vi "Event Handler.vi"(8 "error in (no error)":errorcluster, 10 "Stop Event Handler":refnum<user-event>, 11 "TreeSelection in":refnum<class "TreeSelection.lvclass">) -> (0 "error out":errorcluster)   [LabVIEW 2015, in "TreeSelection.lvclass"]
doc: "The <b>Event Handler VI</b> is a dynamic dispatch VI that should be overwritten if events are needed to create the enhanced QControl. \n\nBy inheriting from the main Control.lvclass the overwritten <b>Event Handler VI</b> will be launched asynchronously in the initialization of the QControl.\n<b> </b> <b> </b>\n©2016 Q Software Innovations, LLC (QSI)\nwritten by Quentin Alldredge\nproduced in LabVIEW 2015\n\nsupport@qsoftwareinnovations.com\nwww.qsoftwareinnovations.com\n\nAll rights reserved.\n\nRedistribution and use in source and binary forms, with or without modification, are permitted provided that the following conditions are met:\n\n * Redistributions of source code must retain the above copyright notice, this list of conditions and the following disclaimer.\n * Redistributions in binary form must reproduce the above copyright notice, this list of conditions and the following disclaimer in the documentation and/or other materials provided with the distribution.\n * Neither the name of Q Software Innovations, LLC. nor the names of its contributors may be used to endorse or promote products derived from this software without specific prior written permission.\n\nTHIS SOFTWARE IS PROVIDED BY THE COPYRIGHT HOLDERS AND CONTRIBUTORS \"AS IS\" AND ANY EXPRESS OR IMPLIED WARRANTIES, INCLUDING, BUT NOT LIMITED TO, THE IMPLIED WARRANTIES OF MERCHANTABILITY AND FITNESS FOR A PARTICULAR PURPOSE ARE DISCLAIMED. IN NO EVENT SHALL THE COPYRIGHT OWNER OR CONTRIBUTORS BE LIABLE FOR ANY DIRECT, INDIRECT, INCIDENTAL, SPECIAL, EXEMPLARY, OR CONSEQUENTIAL DAMAGES (INCLUDING, BUT NOT LIMITED TO, PROCUREMENT OF SUBSTITUTE GOODS OR SERVICES; LOSS OF USE, DATA, OR PROFITS; OR BUSINESS INTERRUPTION) HOWEVER CAUSED AND ON ANY THEORY OF LIABILITY, WHETHER IN CONTRACT, STRICT LIABILITY, OR TORT (INCLUDING NEGLIGENCE OR OTHERWISE) ARISING IN ANY WAY OUT OF THE USE OF THIS SOFTWARE, EVEN IF ADVISED OF THE POSSIBILITY OF SUCH DAMAGE."
uses:
  TreeSelection.lvclass
  TreeSelection.lvclass/TreeSelection.ctl
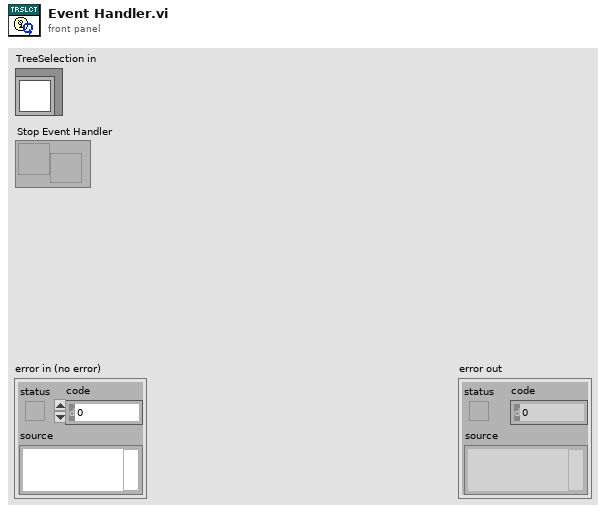
[diagram p1: front panel]
types:
  T1 = typedef "LVPoint32TypeDef.ctl" = cluster{"Horizontal":i32, "Vertical":i32}
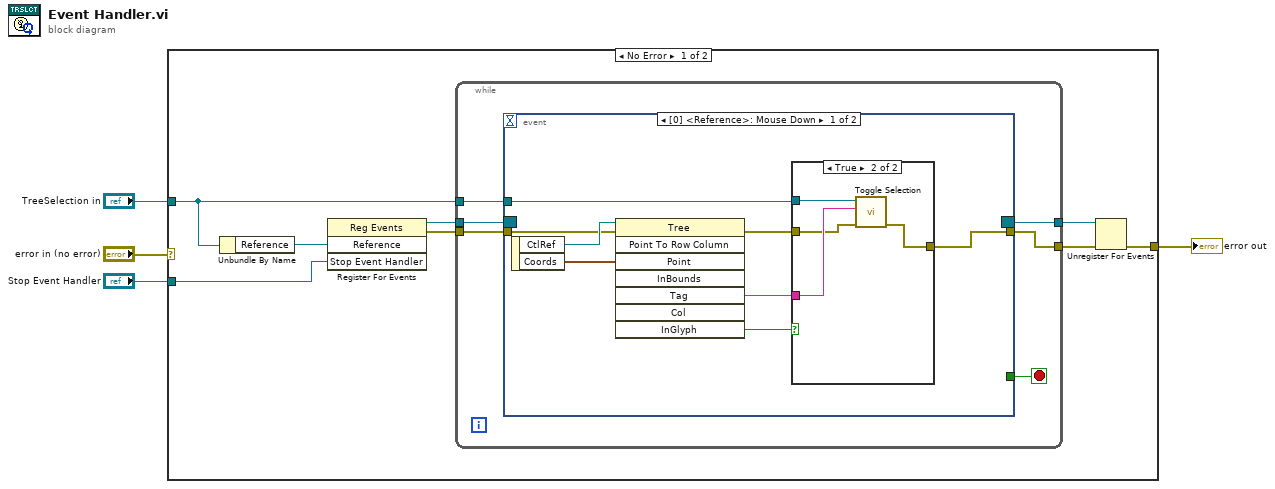
[diagram p0: block diagram]
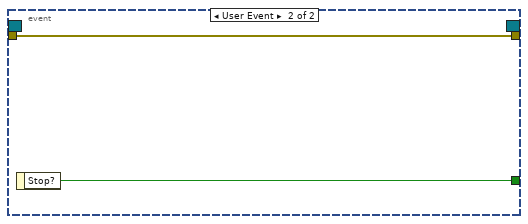
[diagram p3: hidden frame]
diagram:
  n1 = case shown="No Error" "error in (no error)" {
    selector: "error in (no error)" -> [_ w34]
    tunnel: [w9 w34] -> w3
    tunnel: "TreeSelection in" -> [w7 _]
    tunnel: "Stop Event Handler" -> [w5 _]
    frame No Error {
      n2 = Unbundle By Name(w7) -> ("Reference"=w6:refnum<vi>)
      n3 = register-events(w6, w5) -> (reference out=w12:refnum<event-registration>, error out=w11:errorcluster)  [unwired: 2 in]
      n4 = while {
        tunnel: w12 -> [w18]
        tunnel: w11 -> [w16]
        tunnel: [w15] -> w10
        tunnel: [w13] -> w8
        tunnel: w7 -> [w17]
        stop <- w14 stop-if-true
        n5 = event shown="[0] <Reference>: Mouse Down" {
          selector: w18 -> [_ _]
          dyn-events: [_ _] -> w13
          timeout: _ -> [_ _]
          tunnel: w17 -> [w24 _]
          tunnel: w16 -> [w21 w33]
          tunnel: [w19 w33] -> w15
          tunnel: [_ w32] -> w14
          event Mouse Down {
            n6 = event-data() -> ("CtlRef"=w26:refnum<vi>, "Coords"=w25:T1)  [unwired: 1 in]
            n7 = invoke class="Tree" method="Point To Row Column"(reference=w26, error in=w21, "Point"=w25) -> (error out=w20:errorcluster, "Tag"=w23:string, "InGlyph"=w22:bool)  [unwired: 5 in, 5 out]
            n8 = case shown="True" w22 {
              tunnel: w24 -> [_ w30]
              tunnel: w23 -> [_ w31]
              tunnel: w20 -> [w27 w29]
              tunnel: [w27 w28] -> w19
              frame False {
              }
              frame True {
                n9 = call-dynamic "Toggle Selection.vi"("error in (no error)"=w29, "Tag"=w31, "TreeSelection in"=w30) -> ("error out"=w28:errorcluster)  [unwired: 7 in, 1 out]
              }
            }
          }
          event User Event {
            n10 = event-data() -> ("Stop?"=w32:bool)  [unwired: 1 in]
          }
        }
      }
      n11 = Unregister For Events(event registration refnum=w8, error in=w10) -> (error out=w9:errorcluster)
    }
    frame Error {
    }
  }
  "error out" <- w3
